vi "waitForNewResults.vi"(8 "error in (no error)":errorcluster, 11 "Instrument.Lockin in":refnum<class "Instrument.Lockin.lvclass">) -> (0 "error out":errorcluster, 2 "Results (Dictionary)":cluster{"key":string, "value":dbl}[](array[cluster]), 3 "Instrument.Lockin out":refnum<class "Instrument.Lockin.lvclass">)   [LabVIEW 2019, in "Instrument.Lockin.lvclass"]
uses:
  Instrument.Lockin.lvclass
  <userlib>/LevyLab/Instrument Framework/Instrument Types/Lockin/Instrument.LockinAPI.lvclass
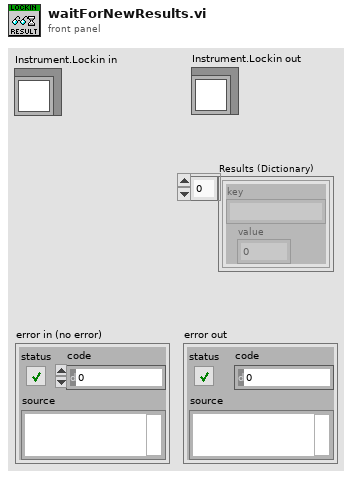
[diagram p1: front panel]
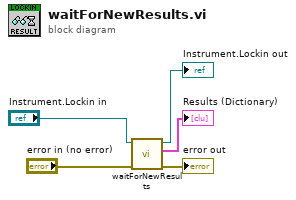
[diagram p0: block diagram]
diagram:
  n1 = call-parent "waitForNewResults.vi"("error in (no error)"="error in (no error)", "Instrument.LockinAPI in"="Instrument.Lockin in") -> ("error out"=→"error out":errorcluster, "Results (Dictionary)"=→"Results (Dictionary)":cluster{"key":string, "value":dbl}[], "Instrument.LockinAPI out"=→"Instrument.Lockin out":refnum<class "Instrument.Lockin.lvclass">)  [unwired: 7 in]
